vi "ASCII Command Tester (Scanning Rig).vi"() -> ()   [LabVIEW 2020]
uses:
  <instrlib>/Arcus Ethernet Driver 1.0.0/ArcusEthernetComm/classes/Controller/_Controller.lvclass
panel:
  out "Home Z":bool
  out "Home Y":bool
  out "Home X":bool
  out "Command 8":bool
  out "Command 7":bool
  out "Command 6":bool
  out "Command 5":bool
  out "Command 4":bool
  out "Command 3":bool
  in  "ASCII Command 8":string
  in  "ASCII Command 7":string
  out "response (out) 8":string
  out "response (out) 7":string
  in  "ASCII Command 6":string
  in  "ASCII Command 5":string
  out "response (out) 6":string
  out "response (out) 5":string
  in  "ASCII Command 4":string
  in  "ASCII Command 3":string
  out "response (out) 4":string
  out "response (out) 3":string
  in  "dev_port(def=5001)":u16=5001
  in  "ip_address (in)":string
  in  "ASCII Command (in)":string
  out "response (out)":string
  out "Command 1":bool
  in  "ASCII Command 2":string
  out "response (out) 2":string
  out "Command 2":bool
  out "Error Out":errorcluster
  in  "Error In":errorcluster
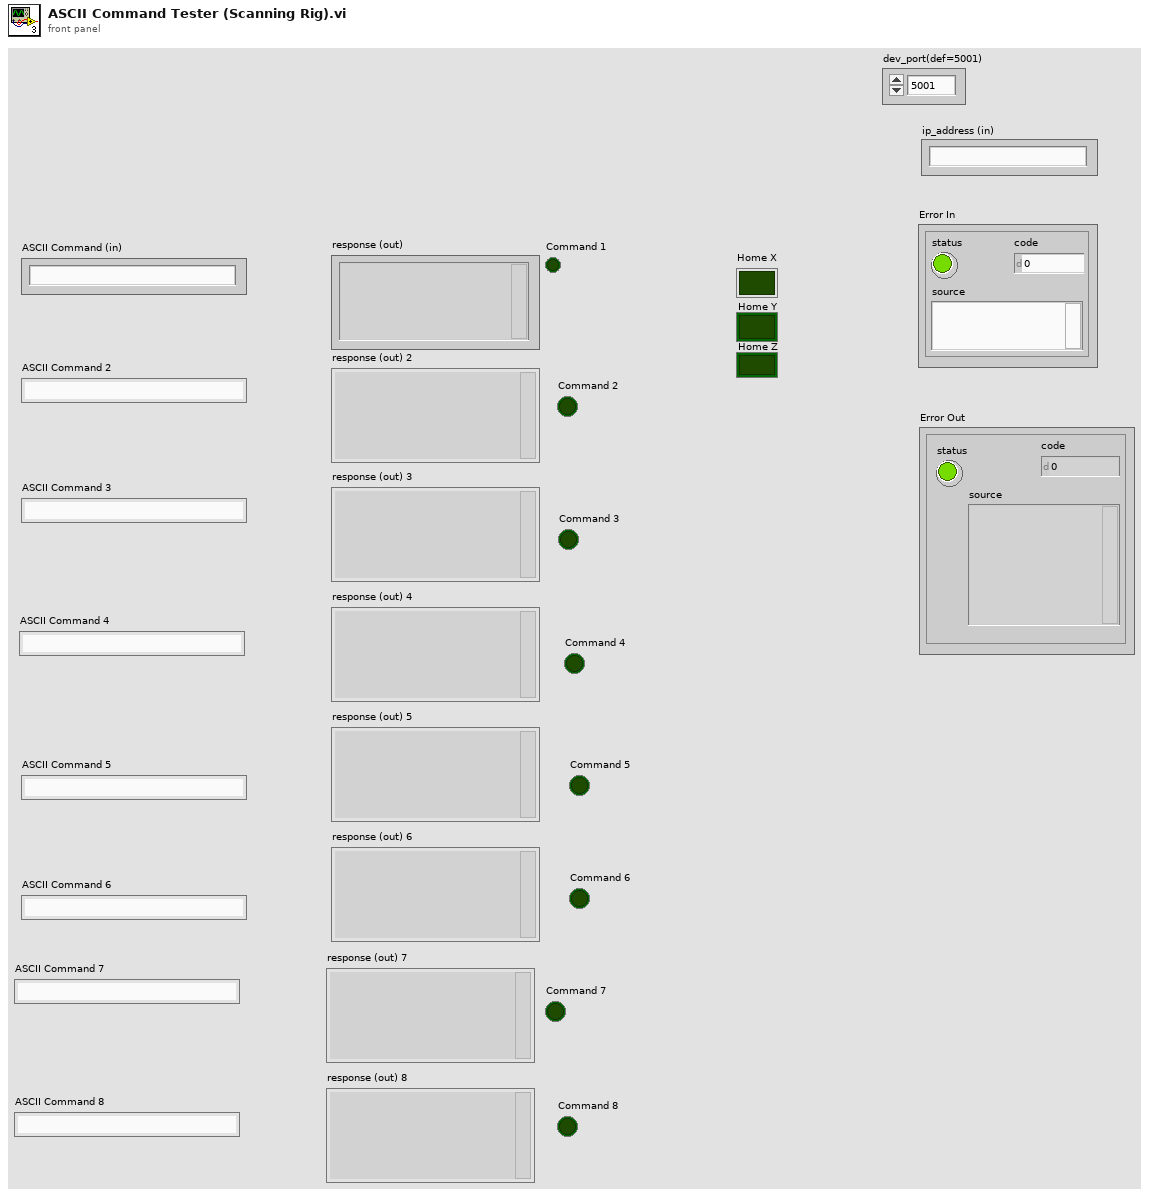
[diagram p1: front panel]
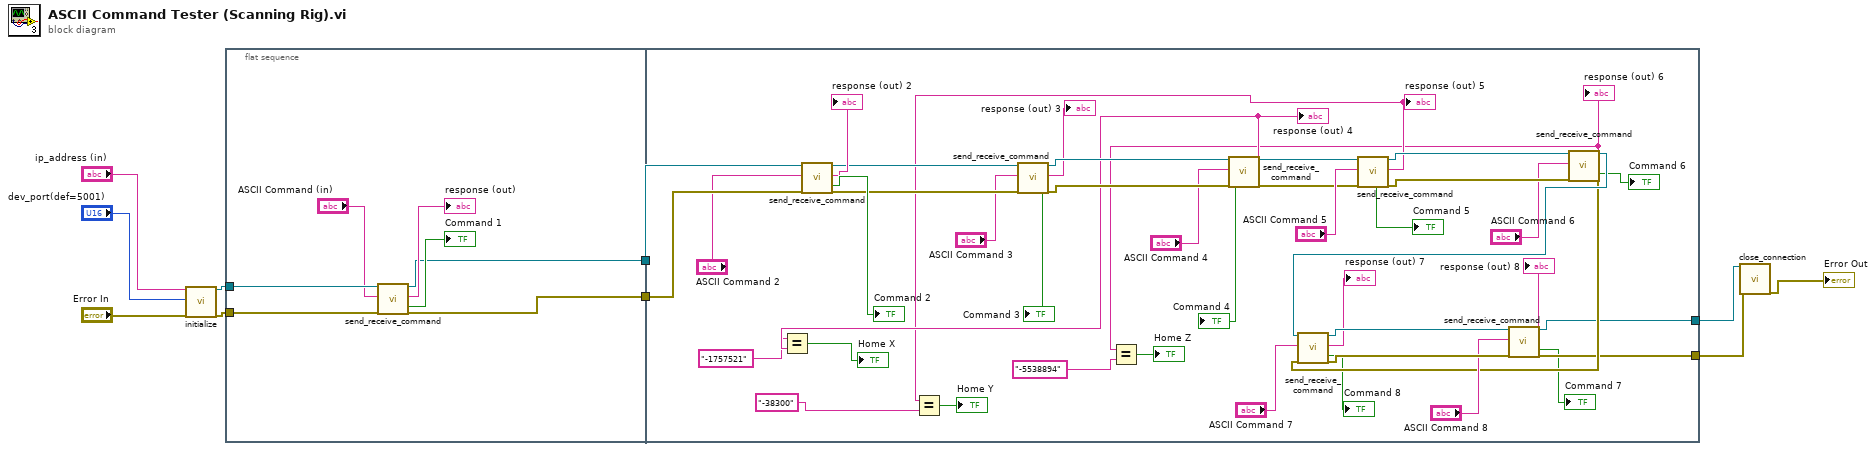
[diagram p0: block diagram]
diagram:
  n1 = call <instrlib>:"initialize.vi"("ip_address (in)"="ip_address (in)", "dev_port(def=5001)"="dev_port(def=5001)", "error in (no error)"="Error In") -> ("reference (out)"=w9:refnum<class "_Controller.lvclass">, "error out"=w8:errorcluster)  [unwired: 15 in]
  n2 = flat-sequence {
    tunnel: w9 -> [w17]
    tunnel: w8 -> [w16]
    tunnel: [w12] -> w5
    tunnel: [w11] -> w4
    tunnel: w5 -> [w60]
    tunnel: w4 -> [w59]
    tunnel: [w28] -> w3
    tunnel: [w35] -> w2
    frame #0 {
      n3 = call <instrlib>:"send_receive_command.vi"("reference (in)"=w17, "ASCII Command (in)"="ASCII Command (in)", "error in (no error)"=w16) -> ("reference (out)"=w12:refnum<class "_Controller.lvclass">, "response (out)"=→"response (out)":string, "success?"=→"Command 1":bool, "error out"=w11:errorcluster)  [unwired: 12 in, 1 out]
    }
    frame #1 {
      n4 = call <instrlib>:"send_receive_command.vi"("reference (in)"=w60, "ASCII Command (in)"="ASCII Command 2", "error in (no error)"=w59) -> ("reference (out)"=w55:refnum<class "_Controller.lvclass">, "response (out)"=→"response (out) 2":string, "success?"=→"Command 2":bool, "error out"=w53:errorcluster)  [unwired: 12 in, 1 out]
      n5 = call <instrlib>:"send_receive_command.vi"("reference (in)"=w55, "ASCII Command (in)"="ASCII Command 3", "error in (no error)"=w53) -> ("reference (out)"=w54:refnum<class "_Controller.lvclass">, "response (out)"=→"response (out) 3":string, "success?"=→"Command 3":bool, "error out"=w52:errorcluster)  [unwired: 12 in, 1 out]
      n6 = call <instrlib>:"send_receive_command.vi"("reference (in)"=w54, "ASCII Command (in)"="ASCII Command 4", "error in (no error)"=w52) -> ("reference (out)"=w26:refnum<class "_Controller.lvclass">, "response (out)"=w25:string, "success?"=→"Command 4":bool, "error out"=w38:errorcluster)  [unwired: 12 in, 1 out]
      "response (out) 4" <- w25
      n7 = Equal?(x="-1757521", y=w25) -> (x = y?=→"Home X":bool)
      n8 = call <instrlib>:"send_receive_command.vi"("reference (in)"=w26, "ASCII Command (in)"="ASCII Command 5", "error in (no error)"=w38) -> ("reference (out)"=w48:refnum<class "_Controller.lvclass">, "response (out)"=w21:string, "success?"=→"Command 5":bool, "error out"=w47:errorcluster)  [unwired: 12 in, 1 out]
      "response (out) 5" <- w21
      n9 = Equal?(x=w21, y="-38300") -> (x = y?=→"Home Y":bool)
      n10 = call <instrlib>:"send_receive_command.vi"("reference (in)"=w48, "ASCII Command (in)"="ASCII Command 6", "error in (no error)"=w47) -> ("reference (out)"=w37:refnum<class "_Controller.lvclass">, "response (out)"=w20:string, "success?"=→"Command 6":bool, "error out"=w36:errorcluster)  [unwired: 12 in, 1 out]
      "response (out) 6" <- w20
      n11 = Equal?(x=w20, y="-5538894") -> (x = y?=→"Home Z":bool)
      n12 = call <instrlib>:"send_receive_command.vi"("reference (in)"=w37, "ASCII Command (in)"="ASCII Command 7", "error in (no error)"=w36) -> ("reference (out)"=w44:refnum<class "_Controller.lvclass">, "response (out)"=→"response (out) 7":string, "success?"=→"Command 8":bool, "error out"=w43:errorcluster)  [unwired: 12 in, 1 out]
      n13 = call <instrlib>:"send_receive_command.vi"("reference (in)"=w44, "ASCII Command (in)"="ASCII Command 8", "error in (no error)"=w43) -> ("reference (out)"=w28:refnum<class "_Controller.lvclass">, "response (out)"=→"response (out) 8":string, "success?"=→"Command 7":bool, "error out"=w35:errorcluster)  [unwired: 12 in, 1 out]
    }
  }
  n14 = call <instrlib>:"close_connection.vi"("reference (in)"=w3, "error in (no error)"=w2) -> ("error out"=→"Error Out":errorcluster)  [unwired: 16 in, 1 out]
